vi "Main.vi"(11 "Module Admin":refnum<class "Delacor_lib_QMH_Cloneable Module Admin.lvclass">) -> ()   [LabVIEW 2026, in "Core.lvlib"]
doc: "This template is based off of the Queued Message Handler design pattern and the Queued Message Handler project template that ships with LabVIEW.\n\nThe main difference is that the queue is private to this module and communication between modules is performed via Broadcast and Request events.\n\nRequest events are wrapped in public API methods and are handled in the Event Handling Loop (EHL) of this VI. Any module can register for Broadcast events sent by this module. The EHL generates messages based on user interface actions.\n\nThe Message Handling Loop (MHL) processes messages generated by the EHL, or by other messages. The messages are string values, so new messages can be added easily to the Message Cases case structure in the MHL. Each message cluster can also provide an optional value for Message Data, which is a variant that can be converted to whatever message-specific data is required.\n_____\nBased on DQMH Dev Tools: Project Template 7.1.2.1547."
uses:
  Core.lvlib
  <vilib>/Delacor/Delacor QMH/Libraries/Cloneable Module Admin_class/Delacor_lib_QMH_Cloneable Module Admin.lvclass
  Module Data--cluster.ctl
  <vilib>/Delacor/Delacor QMH/Libraries/Message Queue_class/Delacor_lib_QMH_Message Queue.lvclass/Delacor_lib_QMH_Message Queue.ctl
  <vilib>/Delacor/Delacor QMH/Libraries/Cloneable Module Admin_class/Delacor_lib_QMH_Cloneable Module Admin.lvclass/Delacor_lib_QMH_Cloneable Module Admin.ctl
  Stop Argument--cluster.ctl
  <vilib>/Delacor/Delacor QMH/Libraries/Module Admin_class/Delacor_lib_QMH_Module Admin.lvclass/Delacor_lib_QMH_Module Admin.ctl
  LaunchEventRecorder Argument--cluster.ctl
  Resubscribe to Cloneable Argument--cluster.ctl
  <vilib>/Utility/miscctls.llb/LVPointTypeDef.ctl
  <vilib>/Delacor/Delacor QMH/Libraries/Message Queue_class/Delacor_lib_QMH_Enqueue Message (Single).vi
  <vilib>/Delacor/Delacor QMH/Libraries/Cloneable Module Admin_class/Delacor_lib_QMH_Get Module ID.vi
  <vilib>/Delacor/Delacor QMH/Libraries/Module Admin_class/Delacor_lib_QMH_Get External Launch.vi
  <vilib>/Delacor/Delacor QMH/Libraries/Message Queue_class/Delacor_lib_QMH_Message Queue.lvclass
  UserEventRecorder/UserEventRecorder.lvlib
panel:
  out "error out":errorcluster
  out "Status":string
  in  "Simulate EHL Error":bool
  in  "Simulate MHL Error":bool
  # "Other processes communicate with this Module via its Public API (wrappers for its Request Events).\n\nThis Module communicates with other processes via its Broadcast Events.\nAny process that wants to receive these messages can register for this module's Broadcast events."
  # "This template is for the DQMH framework. See the block diagram for more information on how to use this template."
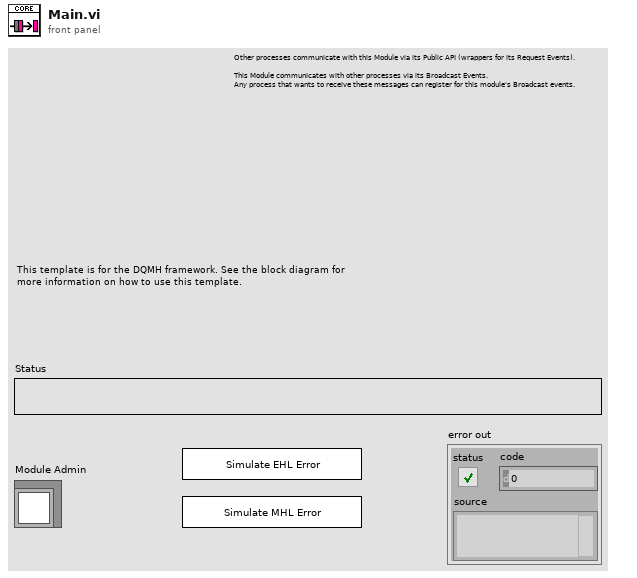
[diagram p1: front panel]
types:
  T1 = typedef "Core.lvlib/Request Events--cluster.ctl" = cluster{"Stop Module":refnum<user-event>, "Show Panel":refnum<user-event>, "Hide Panel":refnum<user-event>, "Show Diagram":refnum<user-event>, "Get Module Execution Status":refnum<user-event>, "LaunchEventRecorder":refnum<user-event>, "Resubscribe to Cloneable":refnum<user-event>}
  T2 = typedef "UserEventRecorder.lvlib/Broadcast Events--cluster.ctl" = cluster{"Module Did Init":refnum<user-event>, "Status Updated":refnum<user-event>, "Error Reported":refnum<user-event>, "Module Did Stop":refnum<user-event>, "Update Module Execution Status":refnum<user-event>}
  T3 = typedef "Core.lvlib/Module Data--cluster.ctl" = cluster{"Status":string, "Module ID Recorder":i32}
  T4 = enum32{"invalid lock state", "Not Locked", "Locked (No Password)", "Password-protected"}
  T5 = typedef "Core.lvlib/Stop Argument--cluster.ctl" = cluster{"Module ID":i32, "Origin":string, "Exit via Stop Module Req?":bool, "Wait for Module to stop?":bool}
  T6 = typedef "Core.lvlib/LaunchEventRecorder Argument--cluster.ctl" = cluster{"Module ID":i32, "Boolean":bool}
  T7 = typedef "Core.lvlib/Resubscribe to Cloneable Argument--cluster.ctl" = cluster{"Module ID":i32, "Boolean":bool}
  T8 = typedef "LVPointTypeDef.ctl" = cluster{"Horizontal":i16, "Vertical":i16}
  T9 = enum32{"Invalid", "Standard", "Closed", "Hidden", "Minimized", "Maximized"}
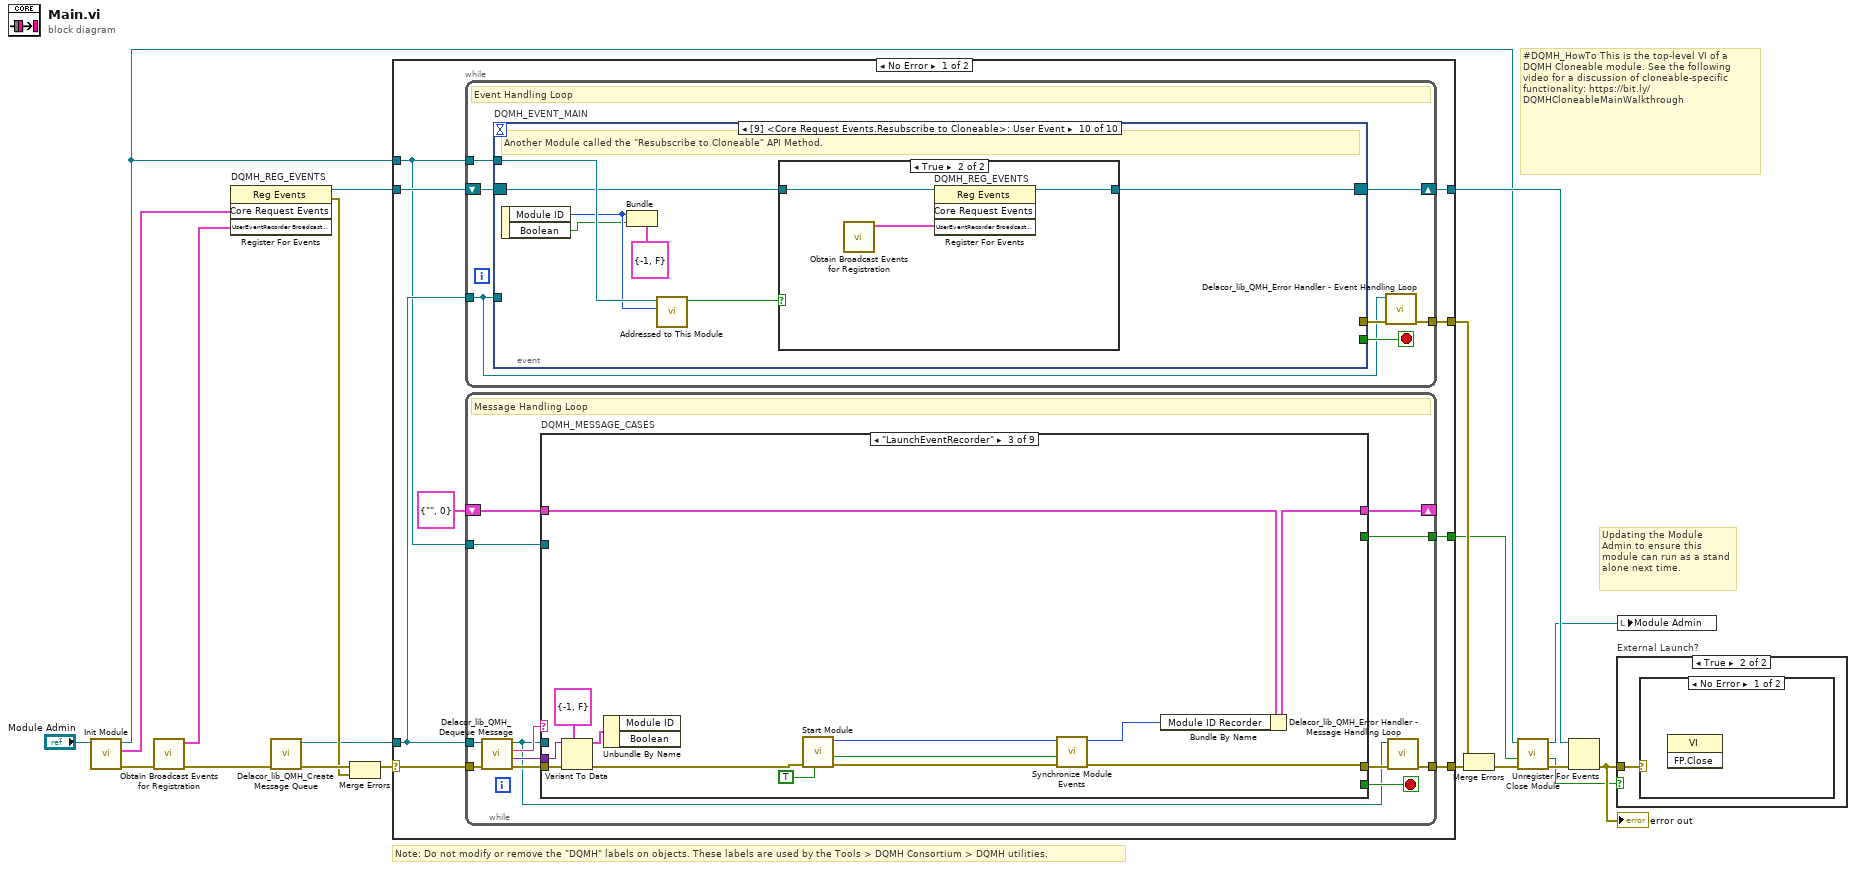
[diagram p0: block diagram]
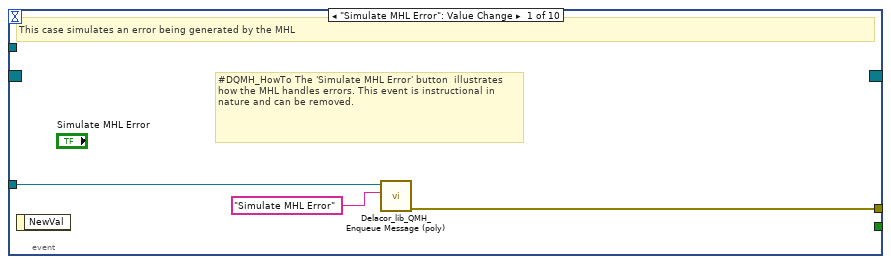
[diagram p2: hidden frame]
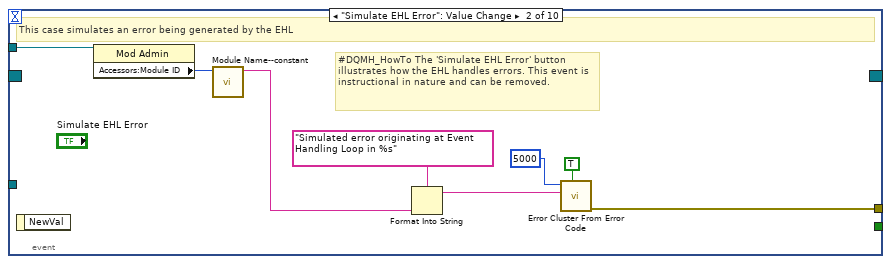
[diagram p3: hidden frame]
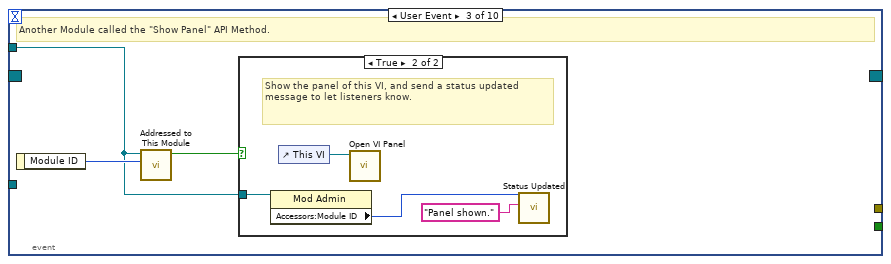
[diagram p4: hidden frame]
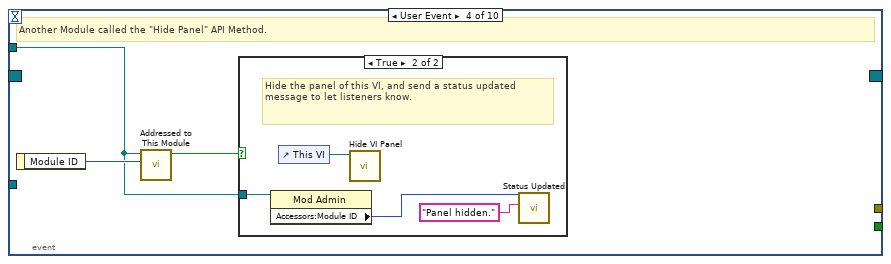
[diagram p6: hidden frame]
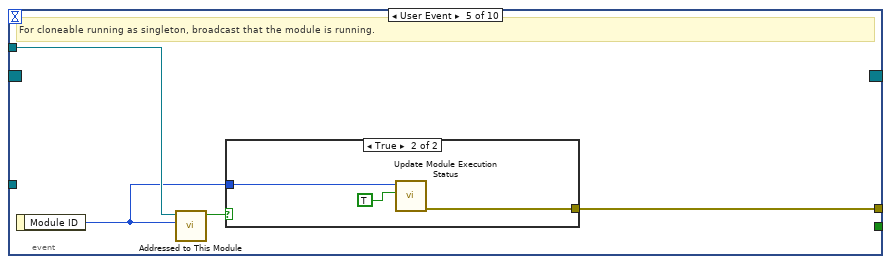
[diagram p8: hidden frame]
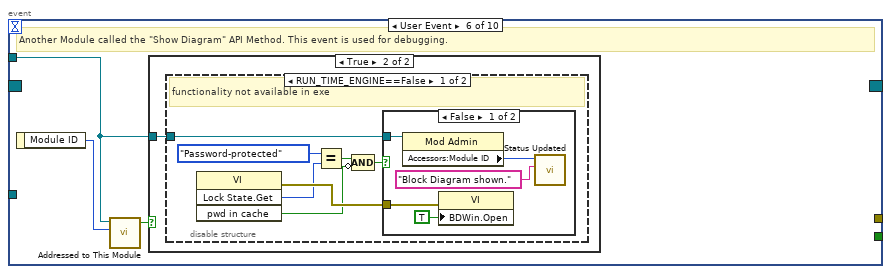
[diagram p10: hidden frame]
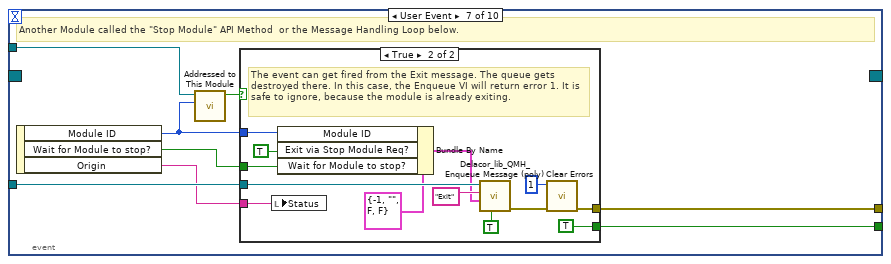
[diagram p14: hidden frame]
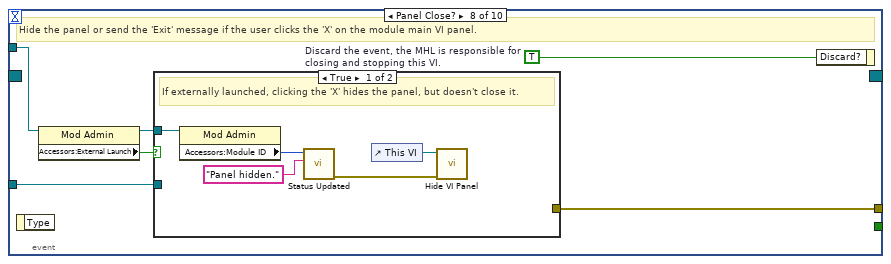
[diagram p16: hidden frame]
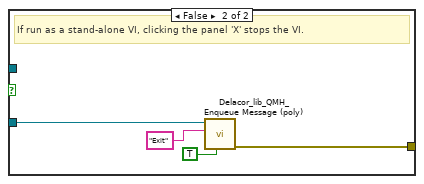
[diagram p17: hidden frame]
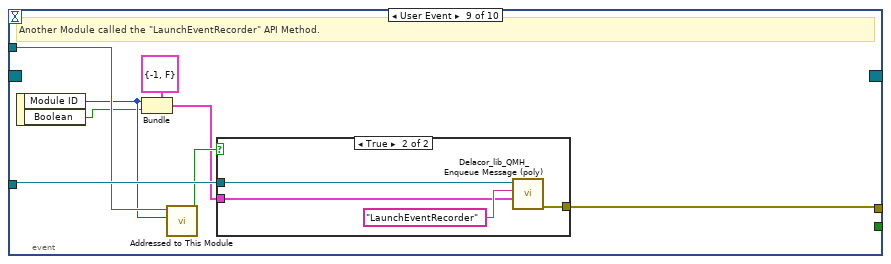
[diagram p18: hidden frame]
diagram:
  # "#DQMH_HowTo This is the top-level VI of a DQMH Cloneable module. See the following video for a discussion of cloneable-specific functionality: https://bit.ly/DQMHCloneableMainWalkthrough"
  # "Note: Do not modify or remove the \"DQMH\" labels on objects. These labels are used by the Tools > DQMH Consortium > DQMH utilities."
  # "Updating the Module Admin to ensure this module can run as a stand alone next time."
  n1 = call "Init Module.vi"("Cloneable Module Admin in"="Module Admin") -> ("error out"=w3:errorcluster, "Core Request Events"=w10:T1, "Cloneable Module Admin out"=w7:refnum<class "Delacor_lib_QMH_Cloneable Module Admin.lvclass">)  [unwired: 8 in]
  n2 = call "Obtain Broadcast Events for Registration.vi"("error in"=w3) -> ("error out"=w2:errorcluster, "UserEventRecorder Broadcast Events"=w1:T2)  [unwired: 8 in, 1 out]
  n3 = register-events "DQMH_REG_EVENTS"(w10, w1) -> (reference out=w11:refnum<event-registration>, error out=w13:errorcluster)  [unwired: 2 in]
  n4 = call <vilib>:"Delacor_lib_QMH_Create Message Queue.vi"("error in"=w2) -> ("error out"=w15:errorcluster, "Message Queue"=w9:refnum<class "Delacor_lib_QMH_Message Queue.lvclass">)  [unwired: 9 in]
  n5 = Merge Errors(w15, w13) -> (w14:errorcluster)
  n6 = case shown="No Error" w14 {
    selector: w14 -> [w27 w267]
    tunnel: [w29 w266] -> w18
    tunnel: [w26 w265] -> w12
    tunnel: w11 -> [w24 w265]
    tunnel: w9 -> [w23 w258]
    tunnel: [w28 _] -> w19
    tunnel: w7 -> [w22 w261]
    tunnel: [w21 _] -> w5
    frame No Error {
      n7 = while {
        tunnel: w23 -> [w30]
        shift-right: [w33] -> w26
        shift-left: w24 -> [w34]
        tunnel: [w35] -> w28
        tunnel: w22 -> [w31]
        stop <- w32 stop-if-true
        # "Event Handling Loop"
        n8 = event "DQMH_EVENT_MAIN" shown="[9] <Core Request Events.Resubscribe to Cloneable>: User Event" {
          selector: w34 -> [_ _ _ _ _ _ _ _ _ w135]
          dyn-events: [_ _ _ _ _ _ _ _ _ w134] -> w33
          timeout: _ -> [_ _ _ _ _ _ _ _ _ _]
          tunnel: [_ _ _ _ _ _ w88 _ _ _] -> w32
          tunnel: w30 -> [w38 _ _ _ _ _ w91 w108 w128 _]
          tunnel: [w39 w47 _ _ w65 _ w92 w111 w121 _] -> w36
          tunnel: w31 -> [_ w46 w48 w55 w63 w69 w90 w109 w126 w139]
          event "Simulate MHL Error": Value Change {
            # "#DQMH_HowTo The 'Simulate MHL Error' button  illustrates how the MHL handles errors. This event is instructional in nature and can be removed."
            # "This case simulates an error being generated by the MHL"
            n9 = event-data() -> ()  [unwired: 1 in, 1 out]
            n10 = call-poly <vilib>:"Delacor_lib_QMH_Enqueue Message (poly).vi"("Message"="Simulate MHL Error", "Message Queue in"=w38) -> ("error out"=w39:errorcluster)  [unwired: 8 in, 1 out]
          }
          event "Simulate EHL Error": Value Change {
            # "#DQMH_HowTo The 'Simulate EHL Error' button  illustrates how the EHL handles errors. This event is instructional in nature and can be removed."
            # "This case simulates an error being generated by the EHL"
            n11 = event-data() -> ()  [unwired: 1 in, 1 out]
            n12 = property on="Property Node" class="Mod Admin"(reference=w46) -> ("Accessors:Module ID"=w45:i32)  [unwired: 1 in, 2 out]
            n13 = call "Module Name--constant.vi"("Module ID"=w45) -> ("Module Name"=w40:string)  [unwired: 10 in]
            n14 = Format Into String(format string="Simulated error originating at Event Handling Loop in %s", w40) -> (resulting string=w43:string)  [unwired: 2 in, 1 out]
            n15 = call <vilib>:"Error Cluster From Error Code.vi"("show call chain? (False)"=TRUE, "error message (\"\")"=w43, "error code (0)"=5000) -> ("error out"=w47:errorcluster)  [unwired: 6 in]
          }
          event User Event {
            # "Another Module called the \"Show Panel\" API Method."
            n16 = event-data() -> ("Module ID"=w49:i32)  [unwired: 1 in]
            n17 = call "Addressed to This Module.vi"("Module ID from Argument"=w49, "Module Admin"=w48) -> ("Addressed to this instance?"=w50:bool)  [unwired: 8 in, 1 out]
            n18 = case shown="True" w50 {
              tunnel: w48 -> [_ w52]
              frame False {
              }
              frame True {
                # "Show the panel of this VI, and send a status updated message to let listeners know."
                n19 = property on="Property Node" class="Mod Admin"(reference=w52) -> ("Accessors:Module ID"=w51:i32)  [unwired: 1 in, 2 out]
                n20 = control-ref of="This VI"() -> (w54:refnum<vi>)
                n21 = call "Open VI Panel.vi"("VI"=w54) -> ()  [unwired: 10 in, 1 out]
                n22 = call "Status Updated.vi"("Status"="Panel shown." ("format string"), "Module ID"=w51) -> ()  [unwired: 9 in, 1 out]
              }
            }
          }
          event User Event {
            # "Another Module called the \"Hide Panel\" API Method."
            n23 = event-data() -> ("Module ID"=w56:i32)  [unwired: 1 in]
            n24 = call "Addressed to This Module.vi"("Module ID from Argument"=w56, "Module Admin"=w55) -> ("Addressed to this instance?"=w57:bool)  [unwired: 8 in, 1 out]
            n25 = case shown="True" w57 {
              tunnel: w55 -> [_ w59]
              frame False {
              }
              frame True {
                # "Hide the panel of this VI, and send a status updated message to let listeners know."
                n26 = property on="Property Node" class="Mod Admin"(reference=w59) -> ("Accessors:Module ID"=w58:i32)  [unwired: 1 in, 2 out]
                n27 = control-ref of="This VI"() -> (w61:refnum<vi>)
                n28 = call "Hide VI Panel.vi"("VI"=w61) -> ()  [unwired: 10 in, 1 out]
                n29 = call "Status Updated.vi"("Status"="Panel hidden." ("format string"), "Module ID"=w58) -> ()  [unwired: 9 in, 1 out]
              }
            }
          }
          event User Event {
            # "For cloneable running as singleton, broadcast that the module is running."
            n30 = event-data() -> ("Module ID"=w62:i32)  [unwired: 1 in]
            n31 = call "Addressed to This Module.vi"("Module ID from Argument"=w62, "Module Admin"=w63) -> ("Addressed to this instance?"=w64:bool)  [unwired: 8 in, 1 out]
            n32 = case shown="True" w64 {
              tunnel: [_ w68] -> w65
              tunnel: w62 -> [_ w67]
              frame False {
              }
              frame True {
                n33 = call "Update Module Execution Status.vi"("Running?"=TRUE, "Module ID"=w67) -> ("error out"=w68:errorcluster)  [unwired: 9 in]
              }
            }
          }
          event User Event {
            # "Another Module called the \"Show Diagram\" API Method. This event is used for debugging."
            n34 = event-data() -> ("Module ID"=w70:i32)  [unwired: 1 in]
            n35 = call "Addressed to This Module.vi"("Module ID from Argument"=w70, "Module Admin"=w69) -> ("Addressed to this instance?"=w71:bool)  [unwired: 8 in, 1 out]
            n36 = case shown="True" w71 {
              tunnel: w69 -> [_ w72]
              frame False {
              }
              frame True {
                n37 = disable-structure shown="RUN_TIME_ENGINE==False" {
                  disable-tunnel: w72 -> [w73 _]
                  frame condition #0 (active) {
                    # "functionality not available in exe"
                    n38 = invoke on="Invoke Node" class="VI" method="Lock State.Get"() -> (error out=w79:errorcluster, "Get Lock State"=w78:T4, "pwd in cache"=w75:bool)  [unwired: 4 in, 1 out]
                    n39 = Equal?(x=T4."Password-protected", y=w78) -> (x = y?=w76:bool)
                    n40 = Compound Arithmetic op=AND(w76, invert w75) -> (w74:bool)
                    n41 = case shown="False" w74 {
                      tunnel: w79 -> [w84 _]
                      tunnel: w73 -> [w81 _]
                      frame False {
                        n42 = property on="Property Node" class="Mod Admin"(reference=w81) -> ("Accessors:Module ID"=w80:i32)  [unwired: 1 in, 2 out]
                        n43 = property on="Property Node" class="VI"(error in=w84, "BDWin.Open"=TRUE ("Block Diagram Window:Open")) -> ()  [unwired: 1 in, 2 out]
                        n44 = call "Status Updated.vi"("Status"="Block Diagram shown." ("format string"), "Module ID"=w80) -> ()  [unwired: 9 in, 1 out]
                      }
                      frame True {
                        # "Password-protected VI, and the password is not in the cache. Do not show the diagram."
                      }
                    }
                  }
                  frame condition #1 {
                  }
                }
              }
            }
          }
          event User Event {
            # "Another Module called the \"Stop Module\" API Method  or the Message Handling Loop below."
            n45 = event-data() -> ("Module ID"=w86:i32, "Wait for Module to stop?"=w87:bool, "Origin"=w85:string)  [unwired: 1 in]
            n46 = call "Addressed to This Module.vi"("Module ID from Argument"=w86, "Module Admin"=w90) -> ("Addressed to this instance?"=w89:bool)  [unwired: 8 in, 1 out]
            n47 = case shown="True" w89 {
              tunnel: [_ w104] -> w92
              tunnel: w91 -> [_ w100]
              tunnel: [_ TRUE] -> w88
              tunnel: w87 -> [_ w95]
              tunnel: w86 -> [_ w97]
              tunnel: w85 -> [_ w93]
              frame False {
              }
              frame True {
                # "The event can get fired from the Exit message. The queue gets destroyed there. In this case, the Enqueue VI will return error 1. It is safe to ignore, because the module is already exiting."
                n48 = local write "Status"(w93) -> ()
                n49 = Bundle By Name(cluster=T5 {"Module ID"=-1, "Origin"="", "Exit via Stop Module Req?"=FALSE, "Wait for Module to stop?"=FALSE} ("Stop Argument"), "Module ID"=w97, "Exit via Stop Module Req?"=TRUE, "Wait for Module to stop?"=w95) -> (w94:T5)
                n50 = call-poly <vilib>:"Delacor_lib_QMH_Enqueue Message (poly).vi"("Priority Message? (F)"=TRUE, "Message Data"=w94, "Message"="Exit", "Message Queue in"=w100) -> ("error out"=w105:errorcluster)  [unwired: 6 in, 1 out]
                n51 = call <vilib>:"Clear Errors.vi"("error in (no error)"=w105, "specific error code to clear (0: all)"=1) -> ("error out"=w104:errorcluster)  [unwired: 4 in, 1 out]
              }
            }
          }
          event Panel Close? {
            w110 = TRUE  # Discard the event, the MHL is responsible for closing and stopping this VI.
            # "Hide the panel or send the 'Exit' message if the user clicks the 'X' on the module main VI panel."
            n52 = event-data() -> ()  [unwired: 1 in, 1 out]
            n53 = property on="Property Node" class="Mod Admin"(reference=w109) -> (reference out=w106:refnum<class "Delacor_lib_QMH_Cloneable Module Admin.lvclass">, "Accessors:External Launch"=w107:bool)  [unwired: 1 in, 1 out]
            n54 = case shown="True" w107 {
              tunnel: w108 -> [_ w119]
              tunnel: [_ w120] -> w111
              tunnel: w106 -> [w114 _]
              frame True {
                # "If externally launched, clicking the 'X' hides the panel, but doesn't close it."
                n55 = property on="Property Node" class="Mod Admin"(reference=w114) -> ("Accessors:Module ID"=w113:i32)  [unwired: 1 in, 2 out]
                n56 = call "Status Updated.vi"("Status"="Panel hidden." ("format string"), "Module ID"=w113) -> ("error out"=w112:errorcluster)  [unwired: 9 in]
                n57 = control-ref of="This VI"() -> (w116:refnum<vi>)
                n58 = call "Hide VI Panel.vi"("error in"=w112, "VI"=w116) -> ()  [unwired: 9 in, 1 out]
              }
              frame False {
                # "If run as a stand-alone VI, clicking the panel 'X' stops the VI."
                n59 = call-poly <vilib>:"Delacor_lib_QMH_Enqueue Message (poly).vi"("Priority Message? (F)"=TRUE, "Message"="Exit", "Message Queue in"=w119) -> ("error out"=w120:errorcluster)  [unwired: 7 in, 1 out]
              }
            }
            n60 = event-data ("Event Filter Node")("Discard?"=w110) -> ()  [unwired: 1 in, 1 out]
          }
          event User Event {
            # "Another Module called the \"LaunchEventRecorder\" API Method."
            n61 = event-data() -> ("Module ID"=w123:i32, "Boolean"=w122:bool)  [unwired: 1 in]
            n62 = Bundle(cluster=T6 {"Module ID"=-1, "Boolean"=FALSE} ("LaunchEventRecorder Argument"), "Module ID"=w123, "Boolean"=w122) -> (w124:T6)
            n63 = call "Addressed to This Module.vi"("Module ID from Argument"=w123, "Module Admin"=w126) -> ("Addressed to this instance?"=w127:bool)  [unwired: 8 in, 1 out]
            n64 = case shown="True" w127 {
              tunnel: w128 -> [_ w132]
              tunnel: w124 -> [_ w130]
              tunnel: [_ w129] -> w121
              frame False {
              }
              frame True {
                n65 = call-poly <vilib>:"Delacor_lib_QMH_Enqueue Message (poly).vi"("Message Data"=w130, "Message"="LaunchEventRecorder", "Message Queue in"=w132) -> ("error out"=w129:errorcluster)  [unwired: 7 in, 1 out]
              }
            }
          }
          event User Event {
            # "Another Module called the \"Resubscribe to Cloneable\" API Method."
            n66 = event-data() -> ("Module ID"=w137:i32, "Boolean"=w136:bool)  [unwired: 1 in]
            n67 = Bundle(cluster=T7 {"Module ID"=-1, "Boolean"=FALSE} ("Resubscribe to Cloneable Argument"), "Module ID"=w137, "Boolean"=w136) -> ()  [unwired: 1 out]
            n68 = call "Addressed to This Module.vi"("Module ID from Argument"=w137, "Module Admin"=w139) -> ("Addressed to this instance?"=w133:bool)  [unwired: 8 in, 1 out]
            n69 = case shown="True" w133 {
              tunnel: w135 -> [w140 w143]
              tunnel: [w140 w141] -> w134
              frame False {
              }
              frame True {
                n70 = call "Obtain Broadcast Events for Registration.vi"() -> ("UserEventRecorder Broadcast Events"=w142:T2)  [unwired: 9 in, 2 out]
                n71 = register-events "DQMH_REG_EVENTS"(reference=w143, w142) -> (reference out=w141:refnum<event-registration>)  [unwired: 2 in, 1 out]
              }
            }
          }
        }
        n72 = call-dynamic "Delacor_lib_QMH_Error Handler - Event Handling Loop.vi"("error in"=w36, "Message Queue in"=w30) -> ("dup error in"=w35:errorcluster)  [unwired: 8 in, 1 out]
      }
      n73 = while {
        tunnel: w23 -> [w144]
        shift-right: [w151] -> _
        shift-left: T3 {"Status"="", "Module ID Recorder"=0} ("Data Cluster") -> [w152]
        tunnel: w27 -> [w155]
        tunnel: [w153] -> w29
        tunnel: w22 -> [w146]
        tunnel: [w145] -> w21
        stop <- w150 stop-if-true
        # "Message Handling Loop"
        n74 = call-dynamic "Delacor_lib_QMH_Dequeue Message.vi"("error in"=w155, "Message Queue in"=w144) -> ("error out"=w154:errorcluster, "Message Data"=w148:variant, "Message"=w149:string, "Message Queue out"=w147:refnum<class "Delacor_lib_QMH_Message Queue.lvclass">)  [unwired: 6 in]
        n75 = case "DQMH_MESSAGE_CASES" shown="\"LaunchEventRecorder\"" w149 {
          selector: w149 -> [_ _ _ _ _ _ _ _ w247]
          tunnel: w147 -> [_ _ _ _ _ w200 _ w239 _]
          tunnel: w154 -> [w175 w179 w192 w195 w197 w209 w226 w245 w256]
          tunnel: [w173 w179 w184 w194 w197 w205 w225 w240 w257] -> w156
          tunnel: w152 -> [w166 w178 w183 w193 w196 w204 w223 w238 w254]
          tunnel: [w165 w178 w182 w193 w196 w204 w223 w238 w254] -> w151
          tunnel: [_ _ _ _ _ _ _ w237 _] -> w150
          tunnel: w148 -> [_ _ w191 _ _ w203 _ w235 _]
          tunnel: w146 -> [w161 _ _ _ _ w202 w221 w230 w253]
          tunnel: [_ _ _ _ _ _ _ w233 _] -> w145
          frame "Initialize" {
            w158 = "Initial Message" ("Initial Message")
            # "#DQMH_CodeNeeded - Initialize the appearance of the front panel."
            # "#DQMH_CodeNeeded - Initialize your state data here."
            # "Initialize - Any operation that needs to be done before the module can receive messages. Synchronize Caller Events.vi will inform Start Module.vi that the module has launched and is ready to receive messages. Module Did Init.vi will broadcast that the module initialized."
            n76 = call "Synchronize Caller Events.vi"("error in"=w175, "Module Admin"=w161) -> ("error out"=w174:errorcluster, "Module Admin out"=w160:refnum<class "Delacor_lib_QMH_Cloneable Module Admin.lvclass">)  [unwired: 8 in]
            n77 = property on="Property Node" class="Mod Admin"(reference=w160) -> ("Accessors:Module ID"=w157:i32, "Accessors:External Launch"=w162:bool)  [unwired: 1 in, 2 out]
            n78 = call "Module Name--constant.vi"("Module ID"=w157) -> ("Module Name"=w170:string)  [unwired: 10 in]
            n79 = property on="Property Node" class="VI"("Front Panel.Title"=w170) -> (reference out=w172:refnum<vi>, error out=w177:errorcluster)  [unwired: 2 in]
            n80 = Select(t=T9."Hidden" ("State"), s=w162, f=T9."Standard" ("State")) -> (s? t:f=w167:T9)
            n81 = invoke on="Invoke Node" class="VI" method="FP.Open"(reference=w172, error in=w177, "State"=w167) -> (reference out=w171:refnum<vi>, error out=w176:errorcluster)  [unwired: 2 in, 3 out]
            n82 = Bundle By Name(cluster=w166, "Status"=w158) -> (w165:T3)
            n83 = invoke on="Invoke Node" class="VI" method="FP.Center"(reference=w171, error in=w176) -> ()  [unwired: 1 in, 3 out]
            n84 = property on="Pane" class="Pane"("Origin"=T8 {"Horizontal"=0, "Vertical"=0}) -> ()  [unwired: 2 in, 2 out]
            n85 = call "Module Name--constant.vi"("Module ID"=w157) -> ("Module Name"=w163:string)  [unwired: 10 in]
            n86 = call "Module Did Init.vi"("error in"=w174, "Initialized?"=TRUE, "Origin"=w163, "Module ID"=w157) -> ("error out"=w173:errorcluster)  [unwired: 7 in]
            "Status" <- w158
          }
          frame "---Module Specific---" {
            # "Separator -- The following cases handle messages specific to this Module."
          }
          frame "LaunchEventRecorder" {
            n87 = Variant To Data(error in=w192, type=T6 {"Module ID"=-1, "Boolean"=FALSE} ("LaunchEventRecorder Argument"), Variant=w191) -> (data=w189:T6, error out=w185:errorcluster)
            n88 = Unbundle By Name(w189) -> ()  [unwired: 2 out]
            n89 = call "Start Module.vi"("Show Main VI Diagram on Init (F)"=TRUE, "error in"=w185) -> ("error out"=w188:errorcluster, "Wait for Event Sync?"=w187:bool, "Module ID"=w186:i32)  [unwired: 5 in, 2 out]
            n90 = call "Synchronize Module Events.vi"("error in"=w188, "Wait for Event Sync?"=w187, "Module ID in"=w186) -> ("error out"=w184:errorcluster, "Module ID out"=w181:i32)  [unwired: 7 in]
            n91 = Bundle By Name(cluster=w183, "Module ID Recorder"=w181) -> (w182:T3)
          }
          frame "---Copy This Frame---" {
            # "Duplicate this frame when creating new messages.  Change this comment in the duplicated frame to describe this message."
            n92 = Merge Errors(w195) -> (w194:errorcluster)
          }
          frame "---Exit and Error Handling---" {
            # "Separator - the following cases handle errors and exit messages."
          }
          frame "Error" {
            # "#DQMH_CodeRecommended - If the module is running in standalone mode (External Launch = FALSE), this code will pop up an error dialog and call the 'Exit' message if an error occurs. Add more fine-grained error management here."
            # "Error - Check the error message data and respond accordingly. This message is sent by the \"Error Handler\" VIs at the end of each loop in this application."
            n93 = property on="Property Node" class="Mod Admin"(reference=w202) -> ("Accessors:External Launch"=w201:bool, "Accessors:Module ID"=w199:i32)  [unwired: 1 in, 2 out]
            n94 = Variant To Data(error in=w209, type=errorcluster {"status"=FALSE, "code"=0, "source"=""} ("error constant"), Variant=w203) -> (data=w198:errorcluster, error out=w207:errorcluster)
            n95 = local write "error out"(w198) -> ()
            n96 = call "Error Reported.vi"("Error"=w198, "Module ID"=w199) -> ()  [unwired: 9 in, 1 out]
            n97 = case shown="False" w201 {
              tunnel: [w214 _] -> w206
              tunnel: w200 -> [w212 _]
              tunnel: w198 -> [w213 _]
              frame False {
                n98 = disable-structure shown="Default" {
                  disable-tunnel: w213 -> [w215 _]
                  frame condition #0 (active) {
                    # "If the module is running standalone, then pop up an error dialog and call the \"Exit\" message."
                    n99 = call <vilib>:"Simple Error Handler.vi"("error in (no error)"=w215) -> ()  [unwired: 4 in, 5 out]
                  }
                  frame condition #1 {
                    # "To prevent the Simple Error Handler VI from being loaded (e.g. when deploying to a Real-Time target), add the Conditional Disable Symbol \"DQMH_Disable_SEH\" to your project and set it to TRUE."
                  }
                }
                n100 = call-poly <vilib>:"Delacor_lib_QMH_Enqueue Message (poly).vi"("Priority Message? (F)"=TRUE, "Message"="Exit", "Message Queue in"=w212) -> ("error out"=w214:errorcluster)  [unwired: 7 in, 1 out]
              }
              frame True {
                # "If the module was launched externally, calling the Error Reported broadcast VI is the only action performed by the \"Error\" message. The module's caller can then process the error appropriately."
              }
            }
            n101 = Merge Errors(w207, w206) -> (w205:errorcluster)
          }
          frame "Simulate MHL Error" {
            # "#DQMH_HowTo The 'Simulate MHL Error' button  illustrates how the MHL handles errors. This event is instructional in nature and can be removed."
            # "Simulate an error occurring at the MHL"
            n102 = property on="Property Node" class="Mod Admin"(reference=w221) -> ("Accessors:Module ID"=w222:i32)  [unwired: 1 in, 2 out]
            n103 = call "Module Name--constant.vi"("Module ID"=w222) -> ("Module Name"=w217:string)  [unwired: 10 in]
            n104 = Format Into String(format string="Simulated error originating at Message Handling Loop in %s", w217) -> (resulting string=w218:string)  [unwired: 2 in, 1 out]
            n105 = call <vilib>:"Error Cluster From Error Code.vi"("show call chain? (False)"=TRUE, "error message (\"\")"=w218, "error code (0)"=5001) -> ("error out"=w224:errorcluster)  [unwired: 6 in]
            n106 = Merge Errors(w226, w224) -> (w225:errorcluster)
          }
          frame "Exit" {
            w236 = 91  # 91: not all Exit messages will have an argument
            w237 = TRUE  # Stop the VI
            # "Release the message queue reference"
            # "#DQMH_CodeNeeded - Add any required cleanup code here."
            # "Exit - Exit the application."
            n107 = Variant To Data(error in=w245, type=T5 {"Module ID"=-1, "Origin"="", "Exit via Stop Module Req?"=FALSE, "Wait for Module to stop?"=FALSE} ("Stop Argument"), Variant=w235) -> (data=w232:T5, error out=w241:errorcluster)
            n108 = call <vilib>:"Clear Errors.vi"("error in (no error)"=w241, "specific error code to clear (0: all)"=w236) -> ("error out"=w244:errorcluster)  [unwired: 4 in, 1 out]
            n109 = property on="Property Node" class="Mod Admin"(reference=w230) -> ("Accessors:Module ID"=w229:i32)  [unwired: 1 in, 2 out]
            n110 = call "Stop Module.vi"("Module ID"=-1) -> ("error out"=w228:errorcluster)  [unwired: 10 in]
            n111 = control-ref of="This VI"() -> (w231:refnum<vi>)
            n112 = call-dynamic "Delacor_lib_QMH_Release Message Queue.vi"("error in"=w244, "Message Queue"=w239) -> ("error out"=w243:errorcluster)  [unwired: 9 in]
            n113 = call "Handle Exit.vi"("error in"=w228, "Stop Argument"=w232, "Module Admin in"=w230, "VI reference"=w231) -> ("error out"=w242:errorcluster, "Wait for Stop?"=w233:bool)  [unwired: 6 in]
            n114 = Merge Errors(w243, w242) -> (w240:errorcluster)
            n115 = call "Error Reported.vi"("Error"=w240, "Module ID"=w229) -> ()  [unwired: 9 in, 1 out]
          }
          frame Default {
            # "'Default' case only runs if there is a message that isn't defined in any of the other cases.  Output a programming error."
            n116 = property on="Property Node" class="Mod Admin"(reference=w253) -> ("Accessors:Module ID"=w252:i32)  [unwired: 1 in, 2 out]
            n117 = call "Module Name--constant.vi"("Module ID"=w252) -> ("Module Name"=w246:string)  [unwired: 10 in]
            n118 = Format Into String(format string="The invalid message string \"%s\" was received in the Message Handling Loop for module \"%s\".", w247, w246) -> (resulting string=w249:string)  [unwired: 2 in, 1 out]
            n119 = call <vilib>:"Error Cluster From Error Code.vi"("show call chain? (False)"=TRUE, "error message (\"\")"=w249, "error code (0)"=1) -> ("error out"=w255:errorcluster)  [unwired: 6 in]
            n120 = Merge Errors(w256, w255) -> (w257:errorcluster)
          }
        }
        n121 = call-dynamic "Delacor_lib_QMH_Error Handler - Message Handling Loop.vi"("error in"=w156, "Message Queue in"=w147) -> ("dup error in"=w153:errorcluster)  [unwired: 8 in, 1 out]
      }
    }
    frame Error {
      n122 = call "Synchronize Caller Events.vi"("Module Admin"=w261) -> ("Module Admin out"=w260:refnum<class "Delacor_lib_QMH_Cloneable Module Admin.lvclass">)  [unwired: 9 in, 1 out]
      n123 = property on="Property Node" class="Mod Admin"(reference=w260) -> ("Accessors:Module ID"=w259:i32)  [unwired: 1 in, 2 out]
      n124 = call-dynamic "Delacor_lib_QMH_Release Message Queue.vi"("error in"=w267, "Message Queue"=w258) -> ("error out"=w266:errorcluster)  [unwired: 9 in]
      n125 = call "Module Name--constant.vi"("Module ID"=w259) -> ("Module Name"=w264:string)  [unwired: 10 in]
      n126 = Format Into String(format string="An error occurred during initialization. %s is no longer running.", w264) -> (resulting string=w262:string)  [unwired: 2 in, 1 out]
      n127 = call "Error Reported.vi"("Additional Information"=w262, "Error"=w266, "Module ID"=w259) -> ()  [unwired: 8 in, 1 out]
    }
  }
  n128 = Merge Errors(w19, w18) -> (w20:errorcluster)
  n129 = call "Close Module.vi"("error in"=w20, "Wait for stop?"=w5, "Module Admin in"=w7) -> ("error out"=w17:errorcluster, "External Launch"=w4:bool, "Module Admin out"=w6:refnum<class "Delacor_lib_QMH_Cloneable Module Admin.lvclass">)  [unwired: 6 in]
  n130 = Unregister For Events(event registration refnum=w12, error in=w17) -> (error out=w16:errorcluster)
  "error out" <- w16
  n131 = case "External Launch?" shown="True" w4 {
    tunnel: w16 -> [_ w268]
    frame False {
    }
    frame True {
      n132 = case shown="No Error" w268 {
        frame No Error {
          n133 = invoke class="VI" method="FP.Close"() -> ()  [unwired: 3 in, 3 out]
        }
        frame Error {
          n134 = disable-structure shown="Default" {
            frame condition #0 (active) {
              n135 = invoke class="VI" method="FP.Open"("Activate"=TRUE ("Activate?")) -> ()  [unwired: 4 in, 5 out]
            }
            frame condition #1 {
              # "Don't show panel on error if running inside a built EXE."
            }
          }
        }
      }
    }
  }
  n136 = local write "Module Admin"(w6) -> ()
